vi "Write Moves List Notifier.vi"(8 "error in (no error)":errorcluster, 10 "Moves List Notifier":refnum<notifier>, 11 "Burrow in":refnum<class "Burrow.lvclass">) -> (0 "error out":errorcluster, 3 "Burrow out":refnum<class "Burrow.lvclass">)   [LabVIEW 2019, in "23.lvlib" / "Burrow.lvclass"]
uses:
  Burrow.lvclass
  Burrow.lvclass/Burrow.ctl
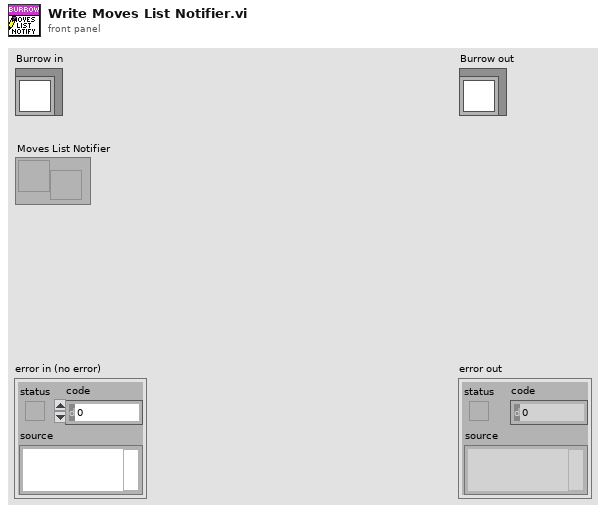
[diagram p1: front panel]
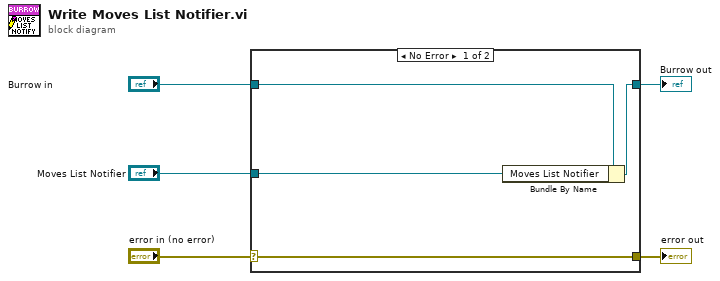
[diagram p0: block diagram]
diagram:
  n1 = case shown="No Error" "error in (no error)" {
    selector: "error in (no error)" -> [w9 w10]
    tunnel: [w9 w10] -> w4
    tunnel: [w7 w11] -> w2
    tunnel: "Burrow in" -> [w8 w11]
    tunnel: "Moves List Notifier" -> [w6 _]
    frame No Error {
      n2 = Bundle By Name(cluster=w8, "Moves List Notifier"=w6) -> (w7:refnum<class "Burrow.lvclass">)
    }
    frame Error {
    }
  }
  "error out" <- w4
  "Burrow out" <- w2
